vi "Oriantation Begin.vi"   [LabVIEW 2013]
uses:
  <vilib>/Rock Robotics/SystemInterfaces/AI/FPGA_AIChannel.ctl
  <vilib>/Rock Robotics/SystemInterfaces/Typedef/FPGA_TypedefAnalogModule.ctl
  <vilib>/Rock Robotics/SystemInterfaces/AI/FPGA_AIGyroChannel.ctl
  <vilib>/Rock Robotics/SystemInterfaces/Typedef/FPGA_TypedefAnalogModuleForGyro.ctl
types:
  T1 = typedef "FPGA_TypedefAnalogModuleForGyro.ctl" = enum16{"Analog Module 1"}
  T2 = typedef "FPGA_AIGyroChannel.ctl" = enum8{"AI 1", "AI 2", "Invalid"}
  T3 = typedef "FPGA_TypedefAnalogModule.ctl" = enum16{"Analog Module 1", "Analog Module 2"}
  T4 = typedef "FPGA_AIChannel.ctl" = enum8{"AI 1", "AI 2", "AI 3", "AI 4", "AI 5", "AI 6", "AI 7", "AI 8", "Invalid"}
  T5 = typedef "WPI_AnalogChannelDevRef.ctl" = cluster{"DevStatus":errorcluster, "Analog Module":T3, "Analog Channel":T4}
  T6 = typedef "WPI_GyroDevRef.ctl" = cluster{"DevStatus":errorcluster, "Analog Module":T3, "Analog Channel":T4, "Offset":dbl, "Gain (VoltsPerDegree/Second)":dbl}
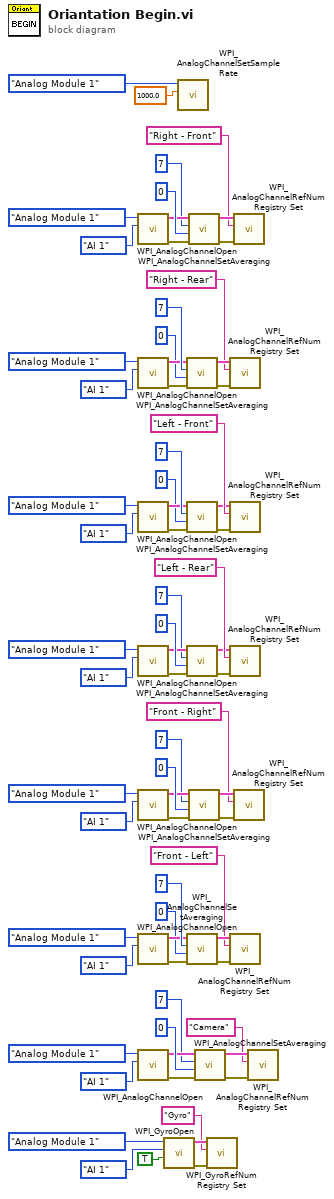
[diagram p0: block diagram]
diagram:
  n1 = call <vilib>:"WPI_AnalogChannelOpen.vi"("Analog Channel"=FPGA_AIChannel."AI 1", "Analog Module (Module 1)"=FPGA_TypedefAnalogModule."Analog Module 1") -> ("error out"=w56:errorcluster, "AIDeviceRef"=w70:T5)  [unwired: 1 in, 7 out]
  n2 = call <vilib>:"WPI_AnalogChannelOpen.vi"("Analog Channel"=FPGA_AIChannel."AI 1", "Analog Module (Module 1)"=FPGA_TypedefAnalogModule."Analog Module 1") -> ("error out"=w57:errorcluster, "AIDeviceRef"=w63:T5)  [unwired: 1 in, 7 out]
  n3 = call <vilib>:"WPI_AnalogChannelOpen.vi"("Analog Channel"=FPGA_AIChannel."AI 1", "Analog Module (Module 1)"=FPGA_TypedefAnalogModule."Analog Module 1") -> ("error out"=w47:errorcluster, "AIDeviceRef"=w35:T5)  [unwired: 1 in, 7 out]
  n4 = call <vilib>:"WPI_AnalogChannelOpen.vi"("Analog Channel"=FPGA_AIChannel."AI 1", "Analog Module (Module 1)"=FPGA_TypedefAnalogModule."Analog Module 1") -> ("error out"=w46:errorcluster, "AIDeviceRef"=w40:T5)  [unwired: 1 in, 7 out]
  n5 = call <vilib>:"WPI_AnalogChannelOpen.vi"("Analog Channel"=FPGA_AIChannel."AI 1", "Analog Module (Module 1)"=FPGA_TypedefAnalogModule."Analog Module 1") -> ("error out"=w20:errorcluster, "AIDeviceRef"=w32:T5)  [unwired: 1 in, 7 out]
  n6 = call <vilib>:"WPI_AnalogChannelOpen.vi"("Analog Channel"=FPGA_AIChannel."AI 1", "Analog Module (Module 1)"=FPGA_TypedefAnalogModule."Analog Module 1") -> ("error out"=w21:errorcluster, "AIDeviceRef"=w27:T5)  [unwired: 1 in, 7 out]
  n7 = call <vilib>:"WPI_AnalogChannelOpen.vi"("Analog Channel"=FPGA_AIChannel."AI 1", "Analog Module (Module 1)"=FPGA_TypedefAnalogModule."Analog Module 1") -> ("error out"=w15:errorcluster, "AIDeviceRef"=w10:T5)  [unwired: 1 in, 7 out]
  n8 = call <vilib>:"WPI_GyroOpen.vi"("Calibrate On Open"=TRUE, "Analog Channel"=FPGA_AIGyroChannel."AI 1", "Analog Module (Module 1)"=FPGA_TypedefAnalogModuleForGyro."Analog Module 1") -> ("error out"=w6:errorcluster, "GyroDevRef"=w5:T6)  [unwired: 6 in, 1 out]
  n9 = call <vilib>:"WPI_AnalogChannelSetSampleRate.vi"("Samples Per Second"=1000.0, "Analog Module (Module 1)"=FPGA_TypedefAnalogModule."Analog Module 1") -> ()  [unwired: 2 in, 8 out]
  n10 = call <vilib>:"WPI_AnalogChannelSetAveraging.vi"("error in (no error)"=w57, "OversampleBits"=u8 0, "AverageBits"=u8 7, "AIDeviceRef"=w63) -> ("error out"=w59:errorcluster, "AIDeviceRef"=w58:T5)  [unwired: 6 out]
  n11 = call <vilib>:"WPI_AnalogChannelSetAveraging.vi"("error in (no error)"=w47, "OversampleBits"=u8 0, "AverageBits"=u8 7, "AIDeviceRef"=w35) -> ("error out"=w48:errorcluster, "AIDeviceRef"=w49:T5)  [unwired: 6 out]
  n12 = call <vilib>:"WPI_AnalogChannelSetAveraging.vi"("error in (no error)"=w46, "OversampleBits"=u8 0, "AverageBits"=u8 7, "AIDeviceRef"=w40) -> ("error out"=w44:errorcluster, "AIDeviceRef"=w45:T5)  [unwired: 6 out]
  n13 = call <vilib>:"WPI_AnalogChannelSetAveraging.vi"("error in (no error)"=w21, "OversampleBits"=u8 0, "AverageBits"=u8 7, "AIDeviceRef"=w27) -> ("error out"=w23:errorcluster, "AIDeviceRef"=w22:T5)  [unwired: 6 out]
  n14 = call <vilib>:"WPI_AnalogChannelSetAveraging.vi"("error in (no error)"=w56, "OversampleBits"=u8 0, "AverageBits"=u8 7, "AIDeviceRef"=w70) -> ("error out"=w55:errorcluster, "AIDeviceRef"=w54:T5)  [unwired: 6 out]
  n15 = call <vilib>:"WPI_AnalogChannelSetAveraging.vi"("error in (no error)"=w20, "OversampleBits"=u8 0, "AverageBits"=u8 7, "AIDeviceRef"=w32) -> ("error out"=w19:errorcluster, "AIDeviceRef"=w18:T5)  [unwired: 6 out]
  n16 = call <vilib>:"WPI_AnalogChannelSetAveraging.vi"("error in (no error)"=w15, "OversampleBits"=u8 0, "AverageBits"=u8 7, "AIDeviceRef"=w10) -> ("error out"=w13:errorcluster, "AIDeviceRef"=w14:T5)  [unwired: 6 out]
  n17 = call <vilib>:"WPI_GyroRefNum Registry Set.vi"("error in (no error)"=w6, "refnum name"="Gyro", "GyroDevRef"=w5) -> ()  [unwired: 7 in, 2 out]
  n18 = call <vilib>:"WPI_AnalogChannelRefNum Registry Set.vi"("error in (no error)"=w59, "refnum name"="Right - Rear", "AIDeviceRef"=w58) -> ()  [unwired: 7 in, 2 out]
  n19 = call <vilib>:"WPI_AnalogChannelRefNum Registry Set.vi"("error in (no error)"=w48, "refnum name"="Left - Front", "AIDeviceRef"=w49) -> ()  [unwired: 7 in, 2 out]
  n20 = call <vilib>:"WPI_AnalogChannelRefNum Registry Set.vi"("error in (no error)"=w44, "refnum name"="Left - Rear", "AIDeviceRef"=w45) -> ()  [unwired: 7 in, 2 out]
  n21 = call <vilib>:"WPI_AnalogChannelRefNum Registry Set.vi"("error in (no error)"=w23, "refnum name"="Front - Left", "AIDeviceRef"=w22) -> ()  [unwired: 7 in, 2 out]
  n22 = call <vilib>:"WPI_AnalogChannelRefNum Registry Set.vi"("error in (no error)"=w55, "refnum name"="Right - Front", "AIDeviceRef"=w54) -> ()  [unwired: 7 in, 2 out]
  n23 = call <vilib>:"WPI_AnalogChannelRefNum Registry Set.vi"("error in (no error)"=w19, "refnum name"="Front - Right", "AIDeviceRef"=w18) -> ()  [unwired: 7 in, 2 out]
  n24 = call <vilib>:"WPI_AnalogChannelRefNum Registry Set.vi"("error in (no error)"=w13, "refnum name"="Camera", "AIDeviceRef"=w14) -> ()  [unwired: 7 in, 2 out]
